vi "Global Data Refs.vi"() -> ()   [LabVIEW 2020, in "Custom Device API.lvlib"]
uses:
  <vilib>/NI VeriStand/Custom Device API/Custom Device API.lvlib
  <vilib>/NI VeriStand/Custom Device API/Data Table Ref.ctl
panel:
  in  "Volt Ref":T1
  in  "Data Ref":T1
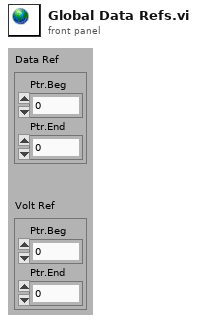
[diagram p1: front panel]
types:
  T1 = typedef "Custom Device API.lvlib/Data Table Ref.ctl" = cluster{"Ptr.Beg":u64, "Ptr.End":u64}
diagram:
